vi "Detection Logic to FPGA Modularized 1Player.vi"() -> ()   [LabVIEW 2026]
uses:
  <vilib>/rvi/Emulation/niFpgaGetClockAttributes.vi
  <vilib>/rvi/Emulation/niFpgaSctlEmulationGetInTimedLoop.vi
  <vilib>/rvi/Emulation/niFpgaEmulationReportErrorSimple.vi
  <extravilib>/ChannelInstances/Tag-bool/Instantiate.vi
  <extravilib>/ChannelInstances/Tag-u8/Instantiate.vi
  <vilib>/rvi/eio/common/nirviEmuTemplateMethod_errors.vi
  <vilib>/rvi/Emulation/niFpgaCriticalErrorInLSC.vi
  <vilib>/eio/EIONode/EIONode.xnode
  <extravilib>/ChannelInstances/Tag-bool.lvlib
  <extravilib>/ChannelInstances/Tag-u8.lvlib
panel:
  in  "Starting Lights":bool[](array[boolean])=[FALSE, FALSE, FALSE, FALSE, FALSE, FALSE, FALSE, FALSE, FALSE, FALSE, FALSE, FALSE, FALSE, FALSE, FALSE, FALSE, FALSE, FALSE, FALSE, FALSE, FALSE, FALSE, FALSE, FALSE, FALSE, FALSE, FALSE, FALSE, FALSE, FALSE, FALSE, FALSE, FALSE, FALSE, FALSE, FALSE, FALSE, FALSE, FALSE, FALSE, FALSE, FALSE, FALSE, FALSE, FALSE]
  out "Time Remaining":u32
  in  "Game Time, uS":u32 caption="Tick Count(uSec)"
  out "Multiplier P1":u16
  out "Random Number":u8
  out "Score P1":u16
  in  "Speed Threshold, ticks":u64=3000
  in  "Debounce Threshold, ticks":u64=1000
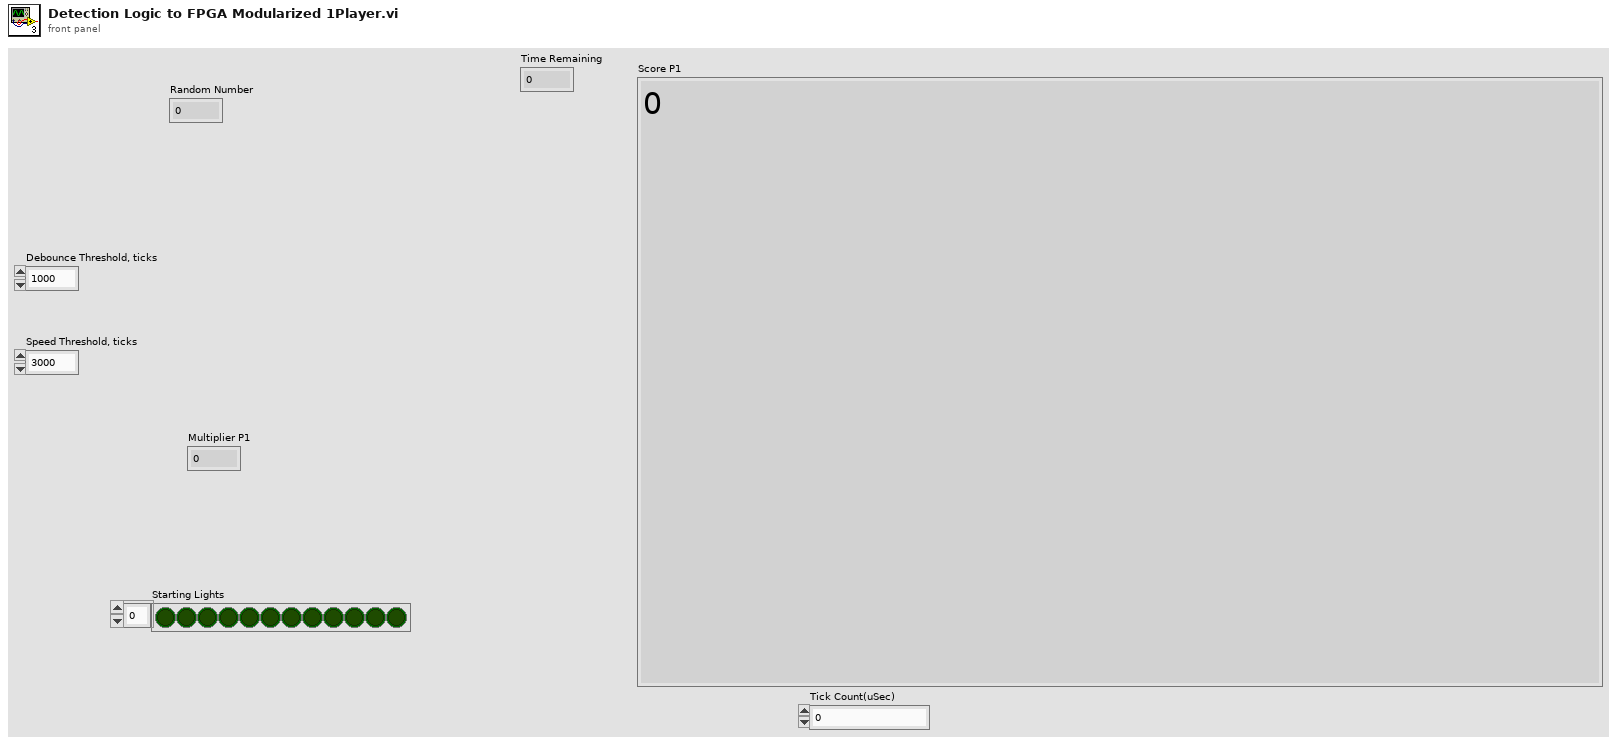
[diagram p1: front panel]
types:
  T1 = cluster{"Score":u16, "Multiplier":u16, "Last Press Tick":u64, u64[]}
  T2 = cluster{"Score out":u16, "Multiplier out":u16, "Last Valid Press Tick out":u64, "Debounce Tick out":u64[]}
  T3 = typedef "Tag-bool.lvlib/))Channel.ctl" = refnum<queue>
  T4 = typedef "Tag-u8.lvlib/))Channel.ctl" = refnum<queue>
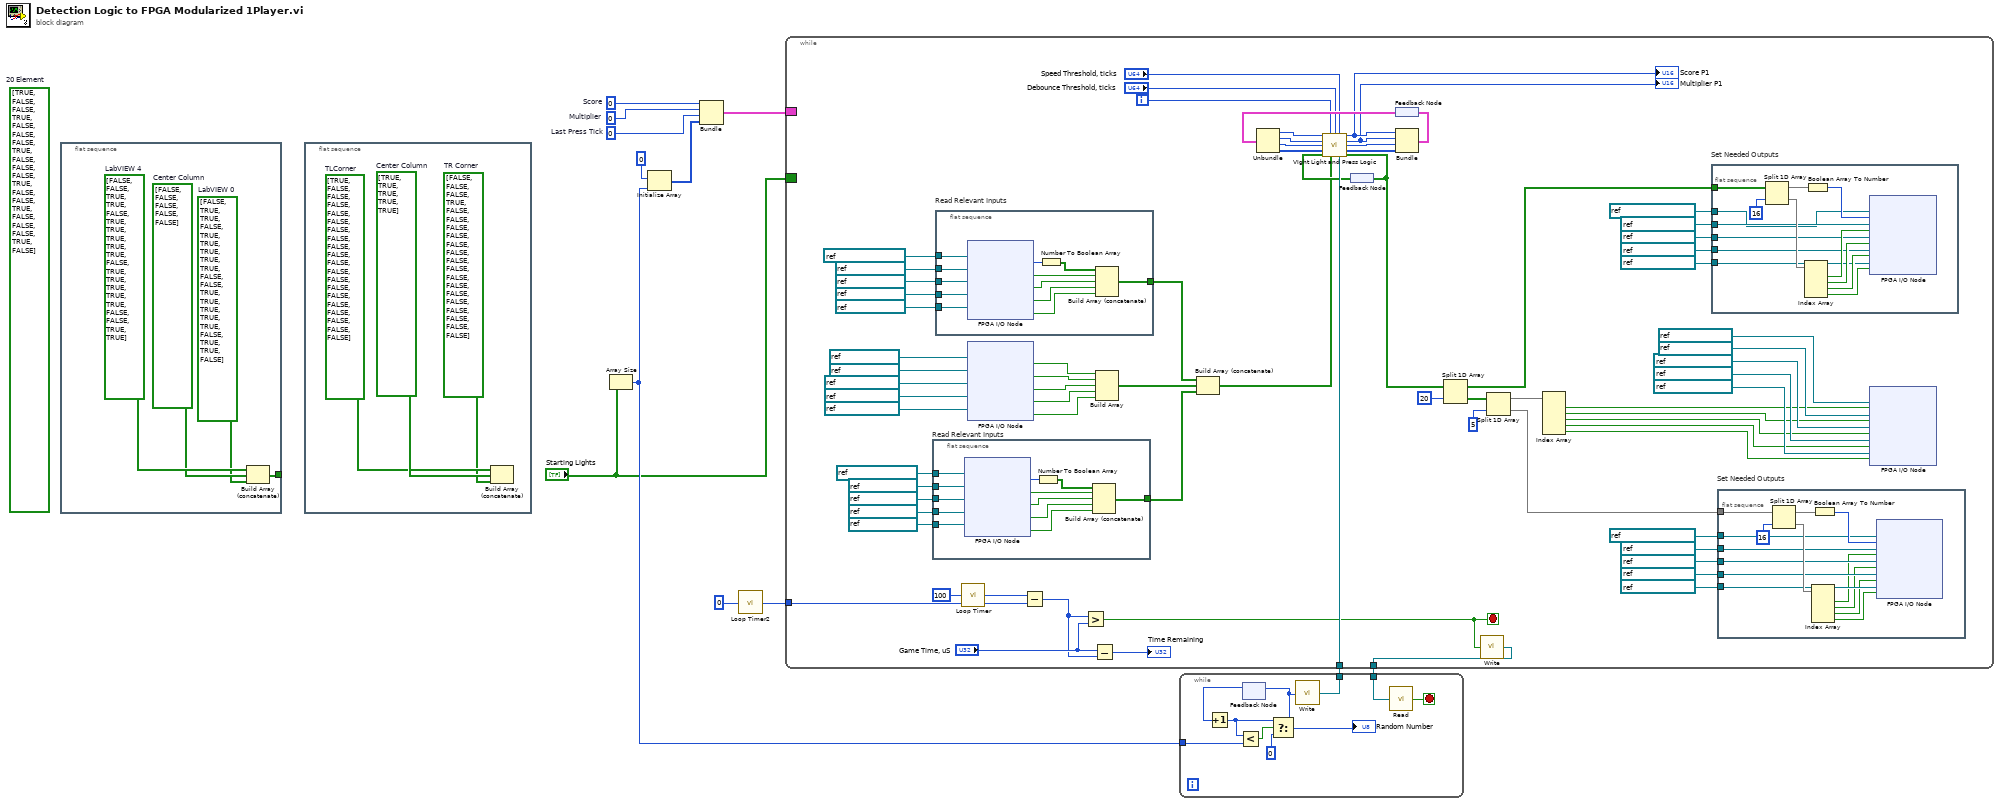
[diagram p0: block diagram]
diagram:
  w8 = u64 0  # Last Press Tick
  (unwired) bool[] [TRUE, FALSE, FALSE, TRUE, FALSE, FALSE, FALSE, TRUE, FALSE, FALSE, FALSE, TRUE, FALSE, FALSE, TRUE, FALSE, FALSE, FALSE, TRUE, FALSE]  # 20 Element
  w9 = u16 0  # Multiplier
  w10 = u16 0  # Score
  n1 = flat-sequence {
    tunnel: [w13] -> _
    frame #0 {
      w15 = bool[] [FALSE, FALSE, FALSE, FALSE, FALSE]  # Center Column
      w14 = bool[] [FALSE, TRUE, TRUE, FALSE, TRUE, TRUE, TRUE, TRUE, TRUE, FALSE, FALSE, TRUE, TRUE, TRUE, TRUE, TRUE, FALSE, TRUE, TRUE, FALSE]  # LabVIEW 0
      w16 = bool[] [FALSE, FALSE, TRUE, TRUE, FALSE, TRUE, TRUE, TRUE, TRUE, TRUE, FALSE, TRUE, TRUE, TRUE, TRUE, TRUE, FALSE, FALSE, TRUE, TRUE]  # LabVIEW 4
      n2 = Build Array (concatenate)(w16, w15, w14) -> (w13:bool[])
    }
  }
  n3 = flat-sequence {
    frame #0 {
      w17 = bool[] [FALSE, FALSE, FALSE, TRUE, FALSE, FALSE, FALSE, FALSE, FALSE, FALSE, FALSE, FALSE, FALSE, FALSE, FALSE, FALSE, FALSE, FALSE, FALSE, FALSE]  # TR Corner
      w19 = bool[] [TRUE, TRUE, TRUE, TRUE, TRUE]  # Center Column
      w18 = bool[] [TRUE, FALSE, FALSE, FALSE, FALSE, FALSE, FALSE, FALSE, FALSE, FALSE, FALSE, FALSE, FALSE, FALSE, FALSE, FALSE, FALSE, FALSE, FALSE, FALSE]  # TLCorner
      n4 = Build Array (concatenate)(w18, w19, w17) -> ()  [unwired: 1 out]
    }
  }
  n5 = Array Size(array="Starting Lights") -> (size(s)=w4:i32)
  n6 = Initialize Array(u64 0 ("Bonus Threshold"), w4) -> (w7:u64[])
  n7 = Bundle("Score"=w10, "Multiplier"=w9, "Last Press Tick"=w8, w7) -> (w6:T1)  [unwired: 1 in]
  n8 = call "Loop Timer2"("Count(uSec)"=u32 0) -> ("Tick Count(uSec)"=w2:u32)
  n9 = while {
    tunnel: [w92] -> w5
    border: "Starting Lights" -> [_]
    tunnel: w11 -> [w93]
    border: w6 -> [_]
    tunnel: w2 -> [w24]
    i -> [w59]
    stop <- w26 stop-if-true
    n10 = flat-sequence "Read Relevant Inputs" {
      tunnel: [w108] -> w55
      tunnel: refnum<k21> "Bank-03/DI7" ("FPGA I/O In") -> [w113]
      tunnel: refnum<k21> "Bank-03/DI6" ("FPGA I/O In") -> [w112]
      tunnel: refnum<k21> "Bank-03/DI5" ("FPGA I/O In") -> [w111]
      tunnel: refnum<k21> "Bank-03/DI4" ("FPGA I/O In") -> [w110]
      tunnel: refnum<k21> "Bank-02/DI15:0" ("FPGA I/O In") -> [w109]
      frame #0 {
        n11 = xnode "FPGA I/O Node"("FPGA I/O In"=w109, "FPGA I/O In"=w110, "FPGA I/O In"=w111, "FPGA I/O In"=w112, "FPGA I/O In"=w113) -> ("I/O Item"=w114:u16, "I/O Item"=w116:bool, "I/O Item"=w117:bool, "I/O Item"=w118:bool, "I/O Item"=w119:bool)  [unwired: 5 out]
        n12 = Number To Boolean Array(number=w114) -> (Boolean array=w115:bool[])
        n13 = Build Array (concatenate)(w115, w116, w117, w118, w119) -> (w108:bool[])
      }
    }
    n14 = flat-sequence "Read Relevant Inputs" {
      tunnel: [w139] -> w56
      tunnel: refnum<k21> "Bank-03/DI3" ("FPGA I/O In") -> [w138]
      tunnel: refnum<k21> "Bank-03/DI2" ("FPGA I/O In") -> [w137]
      tunnel: refnum<k21> "Bank-03/DI1" ("FPGA I/O In") -> [w136]
      tunnel: refnum<k21> "Bank-03/DI0" ("FPGA I/O In") -> [w135]
      tunnel: refnum<k21> "Bank-01/DI15:0" ("FPGA I/O In") -> [w134]
      frame #0 {
        n15 = xnode "FPGA I/O Node"("FPGA I/O In"=w134, "FPGA I/O In"=w135, "FPGA I/O In"=w136, "FPGA I/O In"=w137, "FPGA I/O In"=w138) -> ("I/O Item"=w140:u16, "I/O Item"=w142:bool, "I/O Item"=w143:bool, "I/O Item"=w144:bool, "I/O Item"=w145:bool)  [unwired: 5 out]
        n16 = Number To Boolean Array(number=w140) -> (Boolean array=w141:bool[])
        n17 = Build Array (concatenate)(w141, w142, w143, w144, w145) -> (w139:bool[])
      }
    }
    n18 = call "Loop Timer"("Count(uSec)"=u32 100) -> ("Tick Count(uSec)"=w21:u32)
    n19 = xnode "FPGA I/O Node"("FPGA I/O In"=refnum<k21> "Bank-03/DI8", "FPGA I/O In"=refnum<k21> "Bank-03/DI9", "FPGA I/O In"=refnum<k21> "Bank-03/DI10", "FPGA I/O In"=refnum<k21> "Bank-03/DI11", "FPGA I/O In"=refnum<k21> "Bank-03/DI12") -> ("I/O Item"=w49:bool, "I/O Item"=w48:bool, "I/O Item"=w47:bool, "I/O Item"=w46:bool, "I/O Item"=w45:bool)  [unwired: 5 out]
    n20 = Subtract(x=w21, y=w24) -> (x-y=w20:u32)
    n21 = Greater?(x=w20, y="Game Time, uS") -> (0:w26:bool)
    n22 = Subtract(x="Game Time, uS", y=w20) -> (x-y=→"Time Remaining":u32)
    n23 = Build Array(w49, w48, w47, w46, w45) -> (w44:bool[])
    n24 = Build Array (concatenate)(w56, w44, w55) -> (w43:bool[])
    n25 = feedback #1() -> (w90:bool[])
    n26 = feedback #2() -> (w86:T1)
    n27 = Unbundle(w86) -> ("Score"=w85:u16, "Multiplier"=w84:u16, "Last Press Tick"=w83:u64, w82:u64[])
    n28 = call "VIght Light and Press Logic.vi"("Score in"=w85, "Tick"=w59, "Debounce Threshold, ticks"="Debounce Threshold, ticks", "Speed Threshold, ticks"="Speed Threshold, ticks", "Multiplier in"=w84, "Last Valid Press Tick in"=w83, "Debounce Tick in"=w82, "Lit Buttons"=w90, "Pressed Buttons"=w43, "Random Number"=w93) -> ("Score out"=w81:u16, "Multiplier out"=w80:u16, "Last Valid Press Tick out"=w88:u64, "Debounce Tick out"=w89:u64[], "Buttons to Light"=w40:bool[])  [unwired: 1 in]
    "Score P1" <- w81
    "Multiplier P1" <- w80
    n29 = feedback-in #1(w40) -> ()
    n30 = Bundle("Score out"=w81, "Multiplier out"=w80, "Last Valid Press Tick out"=w88, "Debounce Tick out"=w89) -> (w87:T2)  [unwired: 1 in]
    n31 = feedback-in #2(w87) -> ()
    n32 = Split 1D Array(array=w40, index=20) -> (first subarray=w25:bool[], second subarray=w41:bool[])
    n33 = call <extravilib>:"Write.vi"("element"=w26) -> ("channel"=w92:T3)  [unwired: 1 out]
    n34 = Split 1D Array(array=w41, index=5) -> (first subarray=w32:bool[], second subarray=w38:bool[])
    n35 = Index Array(array=w32) -> (element #1=w31:bool, element #2=w30:bool, element #3=w29:bool, element #4=w28:bool, element #5=w27:bool)  [unwired: 5 in]
    n36 = flat-sequence "Set Needed Outputs" {
      tunnel: w25 -> [w133]
      tunnel: refnum<k21> "Bank-03/DO3" ("FPGA I/O In") -> [w120]
      tunnel: refnum<k21> "Bank-03/DO2" ("FPGA I/O In") -> [w124]
      tunnel: refnum<k21> "Bank-03/DO1" ("FPGA I/O In") -> [w123]
      tunnel: refnum<k21> "Bank-03/DO0" ("FPGA I/O In") -> [w122]
      tunnel: refnum<k21> "Bank-01/DO15:0" ("FPGA I/O In") -> [w121]
      frame #0 {
        n37 = Split 1D Array(array=w133, index=16) -> (first subarray=w131:bool[], second subarray=w129:bool[])
        n38 = Index Array(array=w129) -> (element #1=w128:bool, element #2=w127:bool, element #3=w126:bool, element #4=w125:bool)  [unwired: 4 in]
        n39 = Boolean Array To Number(Boolean array=w131) -> (number=w132:u32)
        n40 = xnode "FPGA I/O Node"("I/O Item"=w132, "FPGA I/O In"=w121, "I/O Item"=w128, "FPGA I/O In"=w122, "I/O Item"=w127, "FPGA I/O In"=w123, "I/O Item"=w126, "FPGA I/O In"=w124, "I/O Item"=w125, "FPGA I/O In"=w120) -> ()  [unwired: 5 out]
      }
    }
    n41 = flat-sequence "Set Needed Outputs" {
      tunnel: refnum<k21> "Bank-03/DO7" ("FPGA I/O In") -> [w101]
      tunnel: refnum<k21> "Bank-03/DO6" ("FPGA I/O In") -> [w104]
      tunnel: refnum<k21> "Bank-03/DO5" ("FPGA I/O In") -> [w103]
      tunnel: refnum<k21> "Bank-03/DO4" ("FPGA I/O In") -> [w102]
      tunnel: refnum<k21> "Bank-02/DO15:0" ("FPGA I/O In") -> [w99]
      tunnel: w38 -> [w100]
      frame #0 {
        n42 = Split 1D Array(array=w100, index=16) -> (first subarray=w98:bool[], second subarray=w105:bool[])
        n43 = Index Array(array=w105) -> (element #1=w97:bool, element #2=w96:bool, element #3=w95:bool, element #4=w94:bool)  [unwired: 4 in]
        n44 = Boolean Array To Number(Boolean array=w98) -> (number=w107:u32)
        n45 = xnode "FPGA I/O Node"("I/O Item"=w107, "FPGA I/O In"=w99, "I/O Item"=w97, "FPGA I/O In"=w102, "I/O Item"=w96, "FPGA I/O In"=w103, "I/O Item"=w95, "FPGA I/O In"=w104, "I/O Item"=w94, "FPGA I/O In"=w101) -> ()  [unwired: 5 out]
      }
    }
    n46 = xnode "FPGA I/O Node"("I/O Item"=w31, "FPGA I/O In"=refnum<k21> "Bank-03/DO8", "I/O Item"=w30, "FPGA I/O In"=refnum<k21> "Bank-03/DO9", "I/O Item"=w29, "FPGA I/O In"=refnum<k21> "Bank-03/DO10", "I/O Item"=w28, "FPGA I/O In"=refnum<k21> "Bank-03/DO11", "I/O Item"=w27, "FPGA I/O In"=refnum<k21> "Bank-03/DO12") -> ()  [unwired: 5 out]
  }
  n47 = while {
    tunnel: w5 -> [w150]
    tunnel: w4 -> [w147]
    tunnel: [w146] -> w11
    stop <- w149 stop-if-true
    n48 = feedback #3() -> (w152:u8)  [unwired: 1 in]
    n49 = Increment(x=w152) -> (x+1=w148:u8)
    n50 = Less?(x=w148, y=w147) -> (x < y?=w153:bool)
    n51 = Select(t=w148, s=w153, f=u8 0) -> (s? t:f=w154:u8)
    "Random Number" <- w154
    n52 = feedback-in #3(w154) -> ()
    n53 = call <extravilib>:"Write.vi"("element"=w154) -> ("channel"=w146:T4)  [unwired: 1 out]
    n54 = call <extravilib>:"Read.vi"("channel"=w150) -> ("element"=w149:bool)  [unwired: 1 in, 1 out]
  }
